vi "Publish Detector Status.vi"(8 "Error In":errorcluster, 11 "KIT-QVA in":refnum<class "KIT-QVA.lvclass">) -> (0 "Error Out":errorcluster, 3 "KIT-QVA out":refnum<class "KIT-QVA.lvclass">)   [LabVIEW 2016, in "KIT-QVA.lvlib" / "KIT-QVA.lvclass"]
doc: "Publish detector status."
uses:
  KIT-QVA.lvclass
  KIT-QVA.lvclass/KIT-QVA.ctl
  CSPP_Core/Classes/CS++ProcessVariables/PVConnection/PVConnection.lvclass/PVConnection.ctl
  CSPP_Core/Classes/CS++ProcessVariables/ProcessVariable/PV.lvclass/PV.ctl
  CSPP_Core/Classes/CS++ProcessVariables/ProcessVariable/Write Data.vi
  CSPP_Core/Classes/CS++ProcessVariables/ProcessVariable/Write Timestamp.vi
  CSPP_Core/Classes/CS++ProcessVariables/ProcessVariable/Write Quality.vi
  CSPP_Core/Classes/CS++ProcessVariables/ProcessVariable/Write status.vi
  CSPP_Core/Classes/CS++ProcessVariables/ProcessVariable/Write Error.vi
  CSPP_Core/Classes/CS++ProcessVariables/ProcessVariable/PV.lvclass
  CSPP_Core/Classes/CS++ProcessVariables/PVConnection/PVConnection.lvclass
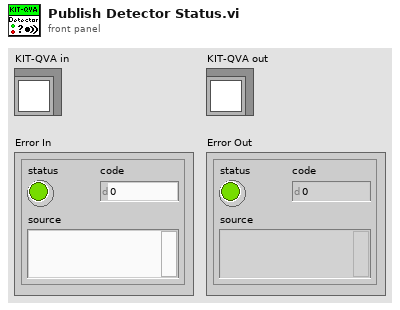
[diagram p1: front panel]
types:
  T1 = cluster{"System Test":bool, "Test Mode":bool, "Fault":bool, "Quench":bool, "U/T Fault":bool, "Bus Error":bool, "System Fault":bool, "Reserved":bool}[]
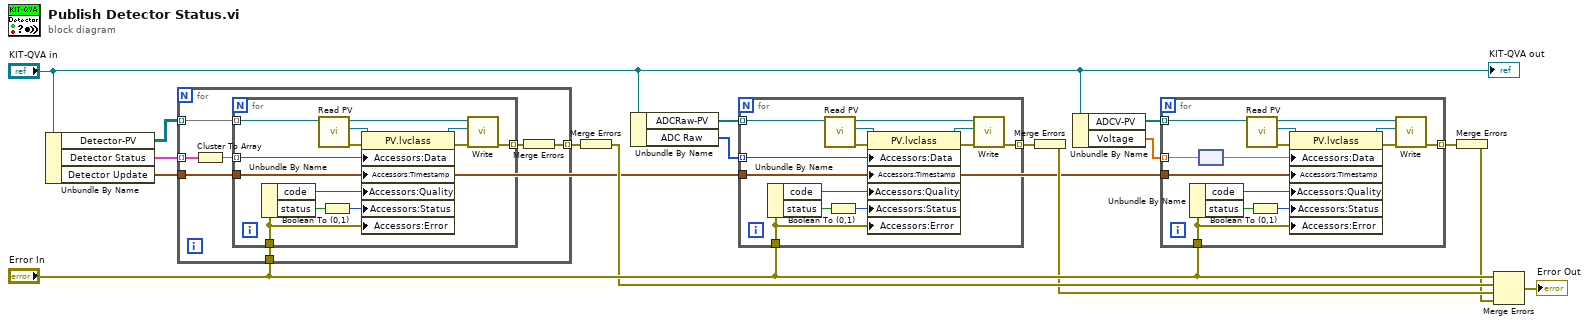
[diagram p0: block diagram]
diagram:
  n1 = Unbundle By Name("KIT-QVA in") -> ("Detector-PV"=w1:refnum<class "PVConnection.lvclass">[][], "Detector Status"=w16:T1, "Detector Update"=w4:timestamp)
  n2 = for {
    tunnel: w1 -> [w23] mode=indexing
    tunnel: "Error In" -> [w22]
    tunnel: [w18] -> w8 mode=indexing
    tunnel: w4 -> [w20]
    tunnel: w16 -> [w19] mode=indexing
    n3 = Cluster To Array(cluster=w19) -> (array=w17:bool[])
    n4 = for {
      tunnel: w17 -> [w28] mode=indexing
      tunnel: w23 -> [w27] mode=indexing
      tunnel: w20 -> [w26]
      tunnel: w22 -> [w25]
      tunnel: [w24] -> w21 mode=indexing
      n5 = Unbundle By Name(w25) -> ("code"=w32:i32, "status"=w31:bool)
      n6 = call "Read PV.vi"("PVConnection in"=w27) -> ("error out"=w30:errorcluster, "PV"=w29:refnum<class "PV.lvclass">, "PVConnection out"=w35:refnum<class "PVConnection.lvclass">)  [unwired: 8 in]
      n7 = Boolean To (0,1)(Boolean=w31) -> (0, 1=w33:i16)
      n8 = property class="PV.lvclass"(reference=w29, error in=w30, "Accessors:Data"=w28, "Accessors:Timestamp"=w26, "Accessors:Quality"=w32, "Accessors:Status"=w33, "Accessors:Error"=w25) -> (reference out=w34:refnum<class "PV.lvclass">, error out=w36:errorcluster)
      n9 = call "Write.vi"("error in (no error)"=w36, "PV"=w34, "PVConnection in"=w35) -> ("error out"=w24:errorcluster)  [unwired: 7 in, 1 out]
    }
    n10 = Merge Errors(w21) -> (w18:errorcluster)
  }
  n11 = Merge Errors(w8) -> (w7:errorcluster)
  n12 = Unbundle By Name("KIT-QVA in") -> ("ADCRaw-PV"=w3:refnum<class "PVConnection.lvclass">[], "ADC Raw"=w15:i16[])
  n13 = for {
    tunnel: w15 -> [w41] mode=indexing
    tunnel: w3 -> [w40] mode=indexing
    tunnel: w4 -> [w39]
    tunnel: "Error In" -> [w38]
    tunnel: [w37] -> w13 mode=indexing
    n14 = Unbundle By Name(w38) -> ("code"=w45:i32, "status"=w44:bool)
    n15 = call "Read PV.vi"("PVConnection in"=w40) -> ("error out"=w43:errorcluster, "PV"=w42:refnum<class "PV.lvclass">, "PVConnection out"=w48:refnum<class "PVConnection.lvclass">)  [unwired: 8 in]
    n16 = Boolean To (0,1)(Boolean=w44) -> (0, 1=w46:i16)
    n17 = property class="PV.lvclass"(reference=w42, error in=w43, "Accessors:Data"=w41, "Accessors:Timestamp"=w39, "Accessors:Quality"=w45, "Accessors:Status"=w46, "Accessors:Error"=w38) -> (reference out=w47:refnum<class "PV.lvclass">, error out=w49:errorcluster)
    n18 = call "Write.vi"("error in (no error)"=w49, "PV"=w47, "PVConnection in"=w48) -> ("error out"=w37:errorcluster)  [unwired: 7 in, 1 out]
  }
  n19 = Merge Errors(w13) -> (w6:errorcluster)
  n20 = Unbundle By Name("KIT-QVA in") -> ("ADCV-PV"=w2:refnum<class "PVConnection.lvclass">[], "Voltage"=w12:dbl[unit][])
  n21 = for {
    tunnel: w12 -> [w55] mode=indexing
    tunnel: w2 -> [w54] mode=indexing
    tunnel: w4 -> [w53]
    tunnel: "Error In" -> [w52]
    tunnel: [w51] -> w10 mode=indexing
    n22 = Unbundle By Name(w52) -> ("code"=w59:i32, "status"=w58:bool)
    n23 = node(w55) -> (w50:dbl)
    n24 = call "Read PV.vi"("PVConnection in"=w54) -> ("error out"=w57:errorcluster, "PV"=w56:refnum<class "PV.lvclass">, "PVConnection out"=w62:refnum<class "PVConnection.lvclass">)  [unwired: 8 in]
    n25 = Boolean To (0,1)(Boolean=w58) -> (0, 1=w60:i16)
    n26 = property class="PV.lvclass"(reference=w56, error in=w57, "Accessors:Data"=w50, "Accessors:Timestamp"=w53, "Accessors:Quality"=w59, "Accessors:Status"=w60, "Accessors:Error"=w52) -> (reference out=w61:refnum<class "PV.lvclass">, error out=w63:errorcluster)
    n27 = call "Write.vi"("error in (no error)"=w63, "PV"=w61, "PVConnection in"=w62) -> ("error out"=w51:errorcluster)  [unwired: 7 in, 1 out]
  }
  n28 = Merge Errors(w10) -> (w5:errorcluster)
  n29 = Merge Errors("Error In", w7, w6, w5) -> (→"Error Out":errorcluster)
  "KIT-QVA out" <- "KIT-QVA in"
